vi "UI_Test.vi"() -> ()   [LabVIEW 2017, in "Client.lvlib"]
uses:
  Client.lvlib
panel:
  out "error out":errorcluster
  out "Connection Quality":dbl(knob) scale=0.0..10.0
  out "Last Update":timestamp
  out "Array":string[](array[string])
  in  "Control Name to update":string
  in  "Tree":string(tree)
  in  "Vertical Stop Button":bool
  in  "Settings":bool
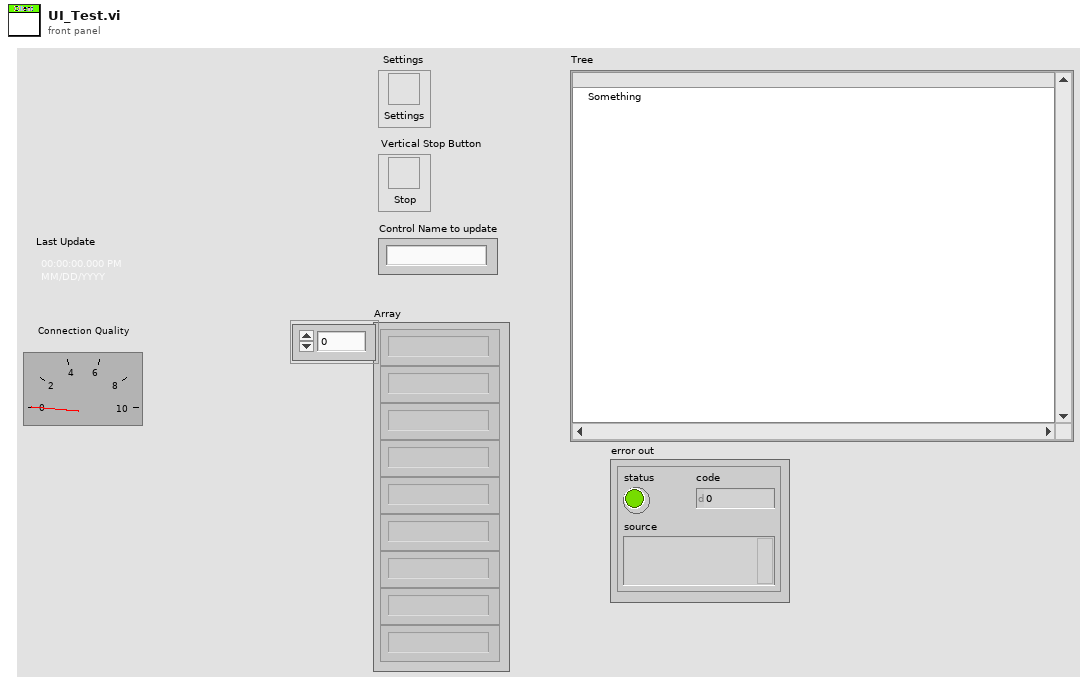
[diagram p1: front panel]
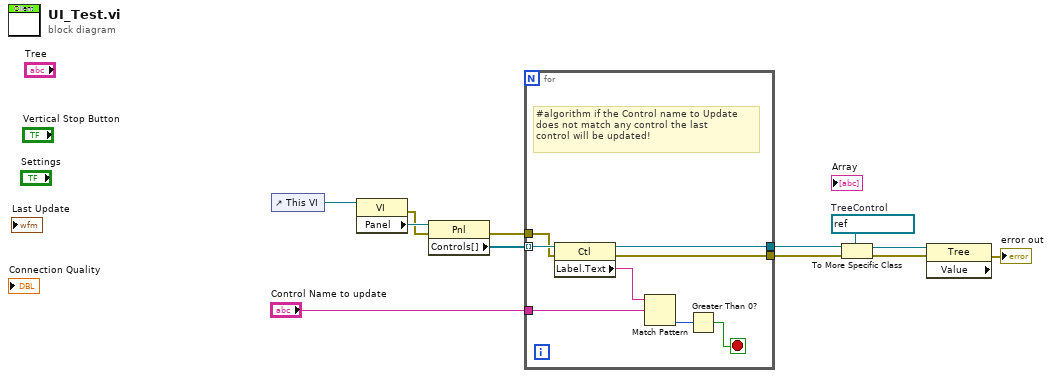
[diagram p0: block diagram]
diagram:
  w7 = refnum<vi> refnum  # TreeControl
  n1 = control-ref of="This VI"() -> (w12:refnum<vi>)
  n2 = property class="VI"(reference=w12) -> (error out=w6:errorcluster, "Panel"=w11:refnum<vi>)  [unwired: 1 in, 1 out]
  n3 = property class="Pnl"(reference=w11, error in=w6) -> (error out=w5:errorcluster, "Controls[]"=w10:refnum<vi>[])  [unwired: 1 out]
  n4 = for {
    tunnel: w10 -> [w16] mode=indexing
    tunnel: "Control Name to update" -> [w20]
    tunnel: [w15] -> w8
    tunnel: w5 -> [w14]
    tunnel: [w13] -> w4
    stop <- w18 stop-if-true
    # "#algorithm if the Control name to Update\ndoes not match any control the last\ncontrol will be updated!"
    n5 = property class="Ctl"(reference=w16, error in=w14) -> (reference out=w15:refnum<vi>, error out=w13:errorcluster, "Label.Text"=w17:string)
    n6 = Match Pattern(string=w17, regular expression=w20) -> (offset past match=w19:i32)  [unwired: 1 in, 3 out]
    n7 = Greater Than 0?(x=w19) -> (x > 0?=w18:bool)
  }
  n8 = To More Specific Class(target class=w7, reference=w8, error in=w4) -> (specific class reference=w3:refnum<vi>, error out=w2:errorcluster)
  n9 = property class="Tree" props=["Value"](reference=w3, error in=w2) -> (error out=→"error out":errorcluster)  [unwired: 2 out]
